vi "Authenticate.vi"(8 "error in (no error)":errorcluster, 9 "Password":string, 10 "Username":string, 11 "Local File Authentication Provider in":refnum<class "Local File Authentication Provider.lvclass">) -> (0 "error out":errorcluster, 2 "User":refnum<class "User.lvclass">, 3 "Local File Authentication Provider out":refnum<class "Local File Authentication Provider.lvclass">)   [LabVIEW 2026, in "Local File Authentication Provider.lvclass"]
uses:
  Local File Authentication Provider.lvclass
  Local File Authentication Provider.lvclass/Local File Authentication Provider.ctl
  Domain/User/User.lvclass
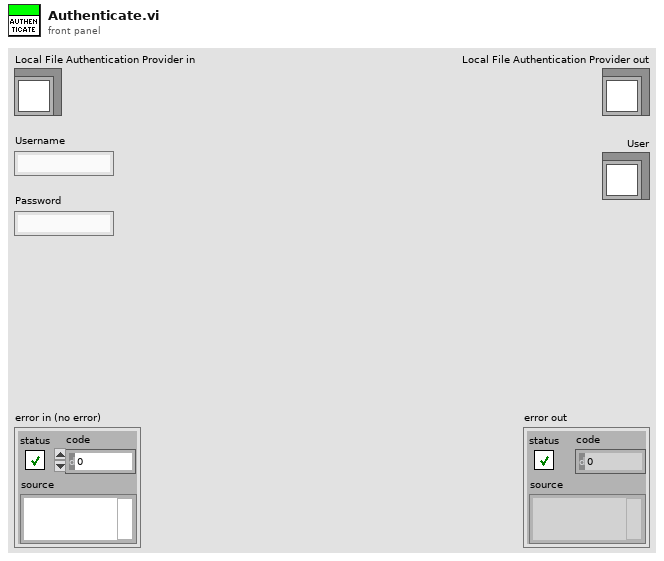
[diagram p1: front panel]
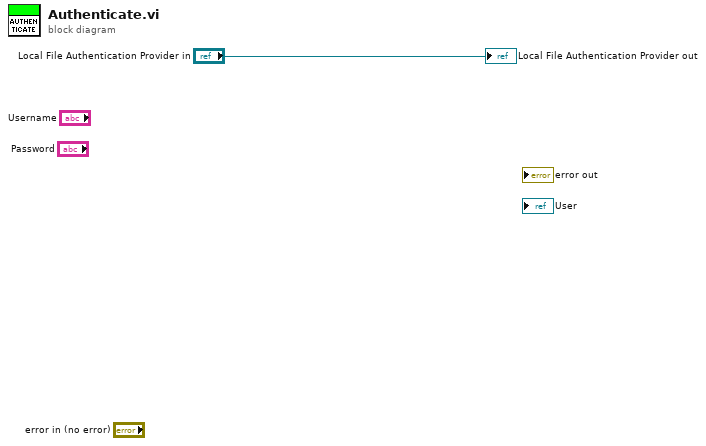
[diagram p0: block diagram]
diagram:
  "Local File Authentication Provider out" <- "Local File Authentication Provider in"
